vi "624FastTalonGetCurrent.vi"(11 "CAN Talon SRX Ref":T1={"DeviceStatus"={"status"=FALSE, "code"=0, "source"=""}, "Type"=enum."PWM", "PWM"={"PWM Channel"=enum."PWM 1", "DeadBand"={"Name"="", "maxPositivePwm"=0, "minPositivePwm"=0, "centerPwm"=0, "maxNegativePwm"=0, "minNegativePwm"=0, "angularRange"=0}}, "CAN"={"Device Number"=0, "Control Mode"=enum."Percent VBus", "Semaphore"=refnum, "Max Vout"=12.0, "TalonSRX Control Mode"=enum."Percent VBus"}, "Invert"=FALSE}) -> (2 "Current":dbl)   [LabVIEW 2015]
uses:
  <vilib>/Rock Robotics/WPI/MotorControl/WPI_MotorControlDeviceRef.ctl
  <vilib>/Rock Robotics/WPI/MotorControl/WPI_MotorControlType.ctl
  <vilib>/Rock Robotics/SystemInterfaces/DIO/FPGA_DIOPWMChannel.ctl
  <vilib>/Rock Robotics/WPI/PWM/WPI_PWMDeadband.ctl
  <vilib>/Rock Robotics/WPI/CAN/Jaguar/SubVIs/WPI_CANJaguar_ControlMode.ctl
  <vilib>/Rock Robotics/WPI/CAN/TalonSRX/WPI_CANTalonSRX_APIControlMode.ctl
  <vilib>/Rock Robotics/WPI/CAN/TalonSRX/WPI_CANTalonSRX_MessageIDs.ctl
panel:
  in  "Device ID (0)":u8
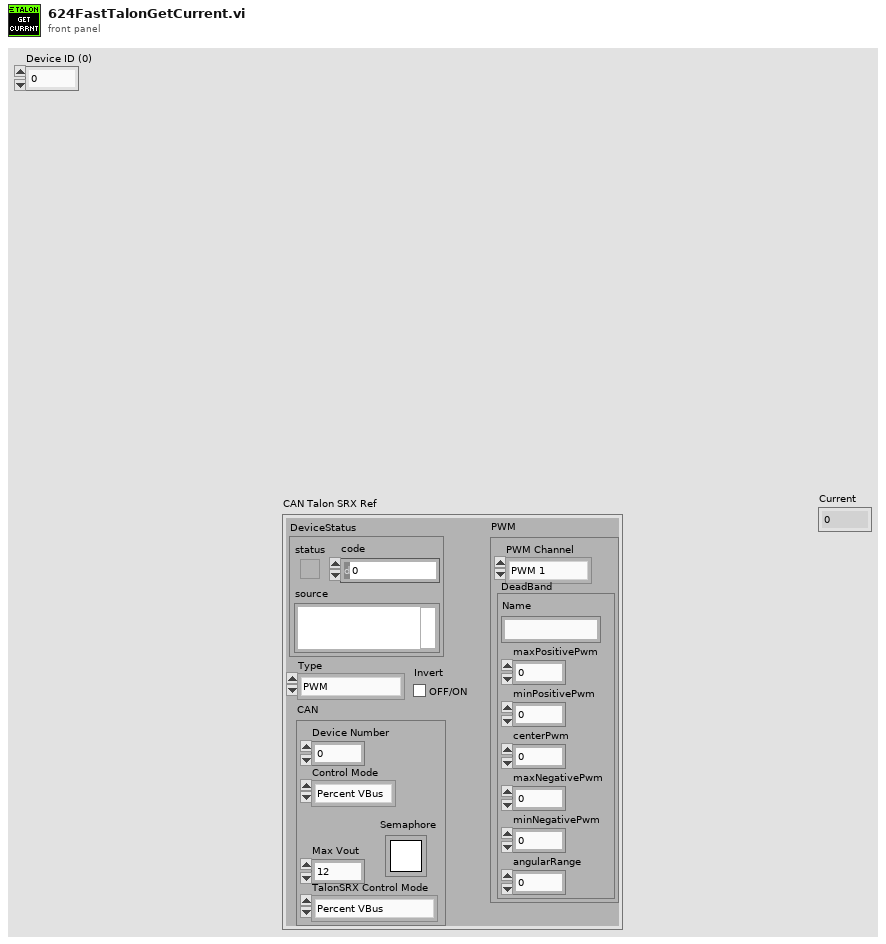
[diagram p1: front panel]
types:
  T1 = typedef "WPI_MotorControlDeviceRef.ctl" = cluster{"DeviceStatus":errorcluster, "Type":T2, "PWM":cluster{"PWM Channel":T3, "DeadBand":T4}, "CAN":cluster{"Device Number":u8, "Control Mode":T5, "Semaphore":T6, "Max Vout":dbl, "TalonSRX Control Mode":T7}, "Invert":bool}
  T2 = typedef "WPI_MotorControlType.ctl" = enum16{"PWM", "CAN", "CANTalonSRX"}
  T3 = typedef "FPGA_DIOPWMChannel.ctl" = enum8{"PWM 0", "PWM 1", "PWM 2", "PWM 3", "PWM 4", "PWM 5", "PWM 6", "PWM 7", "PWM 8", "PWM 9", "PWM MXP 0", "PWM MXP 1", "PWM MXP 2", "PWM MXP 3", "PWM MXP 4", "PWM MXP 5", "PWM MXP 6", "PWM MXP 7", "PWM MXP 8", "PWM MXP 9", "Invalid"}
  T4 = typedef "WPI_PWMDeadband.ctl" = cluster{"Name":string, "maxPositivePwm":i32, "minPositivePwm":i32, "centerPwm":i32, "maxNegativePwm":i32, "minNegativePwm":i32, "angularRange":u16}
  T5 = typedef "WPI_CANJaguar_ControlMode.ctl" = enum8{"Percent VBus", "Current", "Speed", "Position", "Voltage"}
  T6 = typedef "Semaphore RefNum" = refnum<k1>
  T7 = typedef "WPI_CANTalonSRX_APIControlMode.ctl" = enum8{"Percent VBus", "Speed", "Position", "Slave", "Unchanged / Invalid"}
  T8 = typedef "WPI_CANTalonSRX_MessageIDs.ctl" = u32
  T9 = typedef "WPI_CANTalonSRX_GlobalStatus.ctl" = cluster{"Applied Throttle":dbl, "Module Enabled":bool, "CAN Error":errorcluster, "Closed Loop Error":dbl, "Forward Limit Switch Closed":bool, "Reverse Limit Switch Closed":bool, "Sensor Position":dbl, "Sensor Velocity":dbl, "Current":dbl, "Sticky Fault - Over Temp":bool, "Sticky Fault - Under Voltage":bool, "Sticky Fault - Forward Limit":bool, "Sticky Fault - Reverse Limit":bool, "Sticky Fault - Forward Soft Limit":bool, "Sticky Fault - Reverse Soft Limit":bool, "Brake is Enabled":bool, "Encoder Position":dbl, "Encoder Velocity":dbl, "Encoder Index Count":dbl, "Encoder A Pin State":bool, "Encoder B Pin State":bool, "Encoder Index Pin State":bool, "Analog In":dbl, "Analog In Velocity":dbl, "Temperature (C)":dbl, "Battery Voltage":dbl}
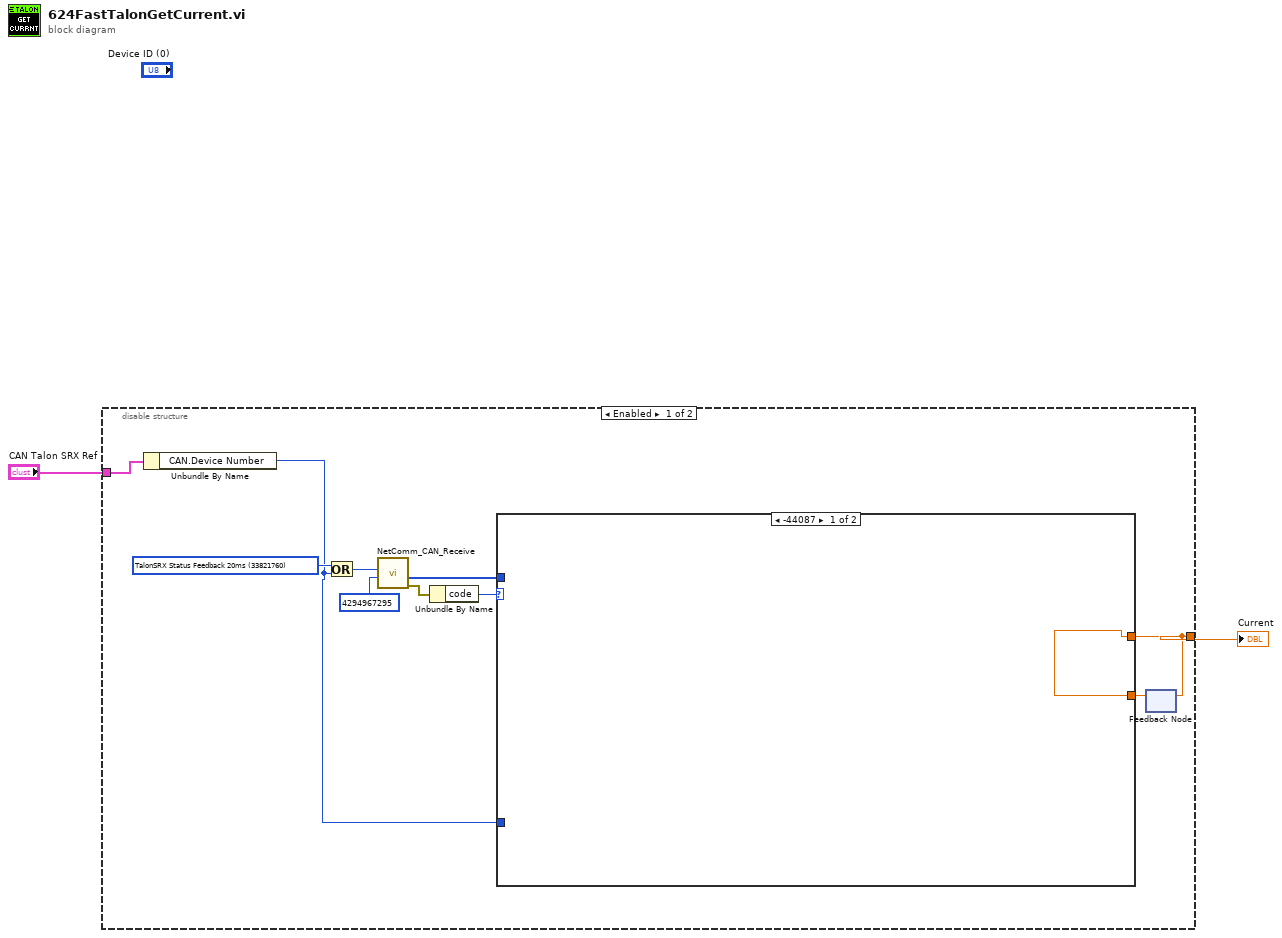
[diagram p0: block diagram]
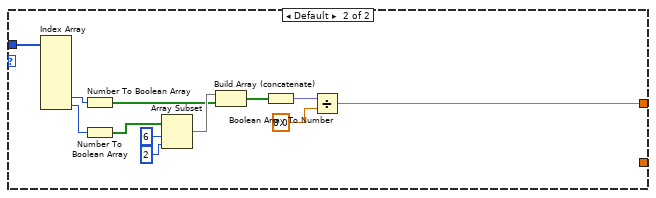
[diagram p2: hidden frame]
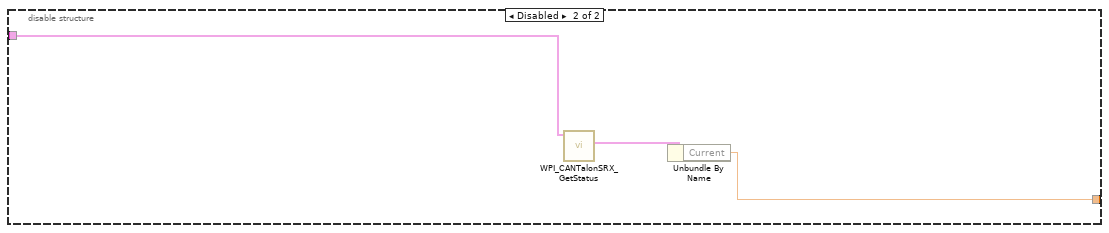
[diagram p3: hidden frame]
diagram:
  n1 = disable-structure shown="Enabled" {
    disable-tunnel: "CAN Talon SRX Ref" -> [w6 w28]
    disable-tunnel: [w4 w26] -> w1
    frame Enabled {
      w9 = T8 33821760 items=["TalonSRX Control General 10ms"=33816576, "TalonSRX Control Rates Slow"=33816640, "TalonSRX Control ClearFlags Slow"=33816704, "TalonSRX Status General 10ms"=33821696, "TalonSRX Status Feedback 20ms"=33821760, "TalonSRX Status Enc 100ms"=33821824, "TalonSRX Status AinTempVbat 100ms"=33821888, "TalonSRX Status Startup Once"=33821952, "TalonSRX Status Debug"=33822080, "TalonSRX Config SetGainsSlot0 A"=33823808, "TalonSRX Config SetGainsSlot0 B"=33823872, "TalonSRX Config SetGainsSlot1 A"=33823936, "TalonSRX Config SetGainsSlot1 B"=33824000, "TalonSRX Config SetSoftLimits"=33824064, "TalonSRX Config WebControl"=33824128, "TalonSRX Param Request"=33822720, "TalonSRX Param Response"=33822784, "TalonSRX Param Set"=33822848]
      n2 = Unbundle By Name(w6) -> ("CAN.Device Number"=w5:u8)
      n3 = Or(x=w9, y=w5) -> (x .or. y?=w8:T8)
      n4 = call <vilib>:"NetComm_CAN_Receive.vi"("Message ID Mask"=u32 4294967295, "Message ID"=w8) -> ("error out"=w11:errorcluster, "Data"=w7:u8[])  [unwired: 6 in, 2 out]
      n5 = Unbundle By Name(w11) -> ("code"=w12:i32)
      n6 = feedback #1() -> (w3:dbl)  [unwired: 1 in]
      n7 = case shown="-44087" w12 {
        tunnel: w5 -> [_ _]
        tunnel: w7 -> [_ w25]
        tunnel: [w13 w14] -> w4
        tunnel: w3 -> [w13 _]
        frame -44087 {
        }
        frame Default {
          n8 = Index Array(array=w25) -> (element #6=w19:u8, element #7=w18:u8)  [unwired: 7 in, 5 out]
          n9 = Number To Boolean Array(number=w19) -> (Boolean array=w15:bool[])
          n10 = Number To Boolean Array(number=w18) -> (Boolean array=w24:bool[])
          n11 = Array Subset(array=w24, index=6, length=2) -> (w16:bool[])
          n12 = Build Array (concatenate)(w16, w15) -> (w22:bool[])
          n13 = Boolean Array To Number(Boolean array=w22) -> (number=w21:fxp<+/-,11,11>)
          n14 = Divide(x=w21, y=8.0) -> (x/y=w14:dbl)
        }
      }
      n15 = feedback-in #1(w4) -> ()
    }
    frame Disabled {
      n16 = call <vilib>:"WPI_CANTalonSRX_GetStatus.vi"("CAN Talon SRX Ref"=w28) -> ("Talon SRX Status"=w27:T9)  [unwired: 8 in, 2 out]
      n17 = Unbundle By Name(w27) -> ("Current"=w26:dbl)
    }
  }
  "Current" <- w1
